vi "Day6Part2.vi"(11 "Input":string="47|53\n97|13\n97|61\n97|47\n75|29\n61|13\n75|53\n29|13\n97|29\n53|29\n61|53\n97|53\n61|29\n47|13\n75|47\n97|75\n47|61\n75|61\n47|29\n75|13\n53|13") -> (3 "Result":i64)   [LabVIEW 2024]
uses:
  <vilib>/Utility/miscctls.llb/LVMapReplaceAction.ctl
  <userlib>/_OpenG.lib/string/string.llb/openg_string.lvlib
panel:
  out "Array":bool[][](array[boolean])
  out "element":string
  out "X":i32
  out "Y":i32
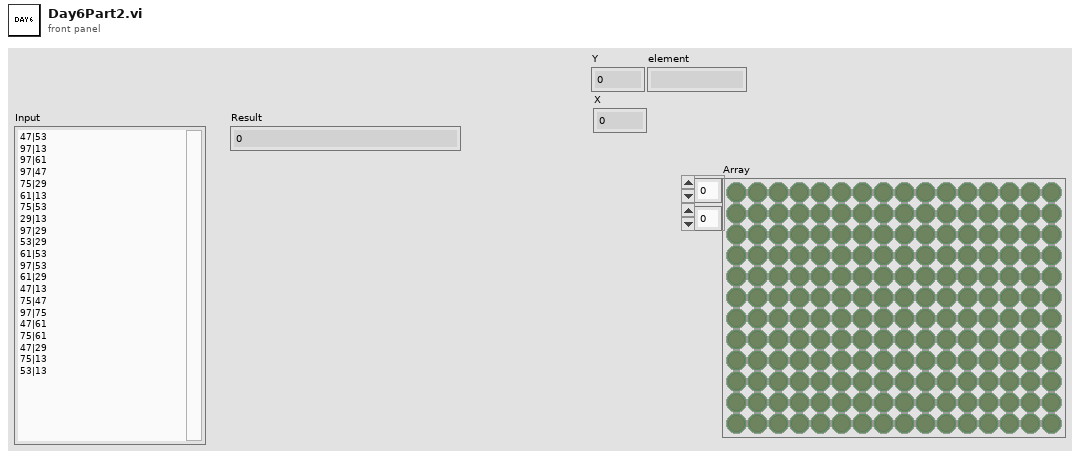
[diagram p1: front panel]
types:
  T1 = typedef "LVMapReplaceAction.ctl" = enum32{"Modify Entry only if found", "Add or Modify Entry", "Delete Entry"}
  T2 = map{cluster{i32, "offset past replacement":i32}, string[]}
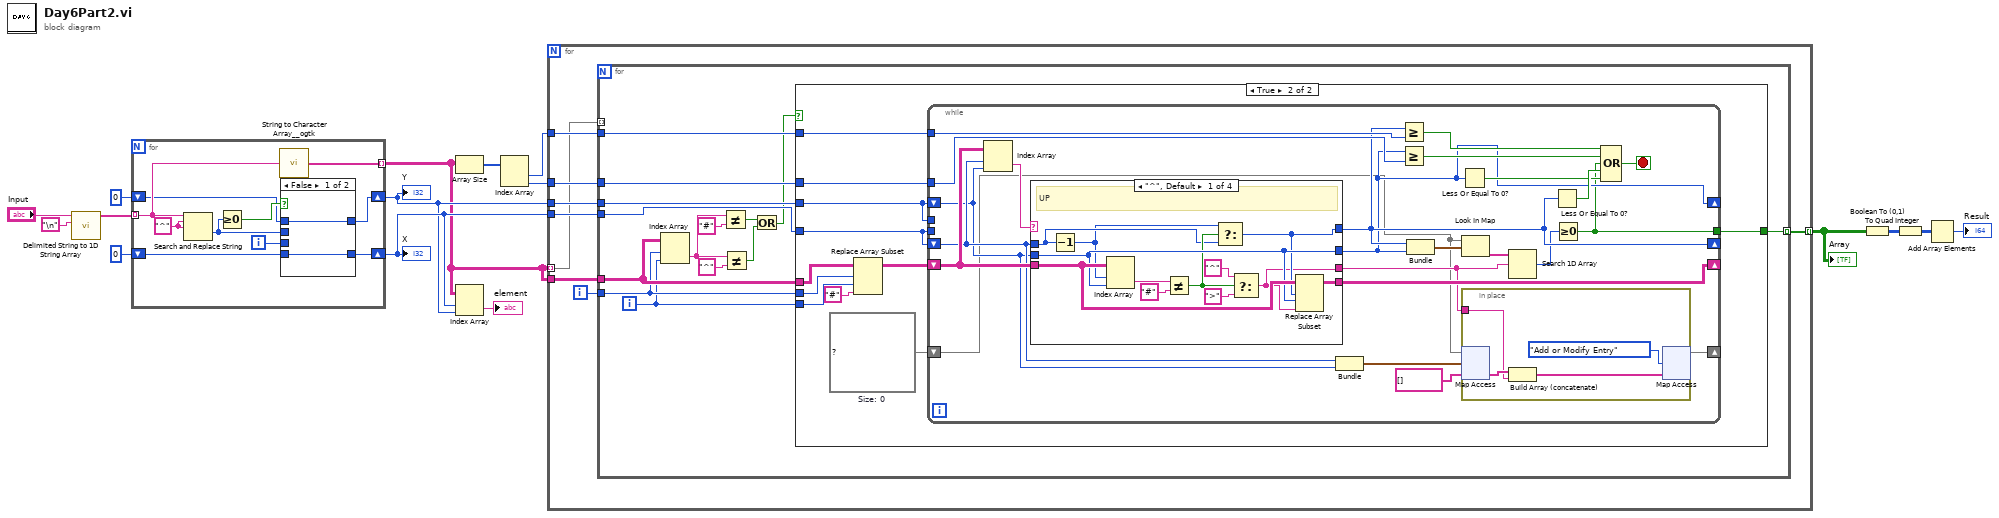
[diagram p0: block diagram]
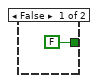
[diagram p2: hidden frame]
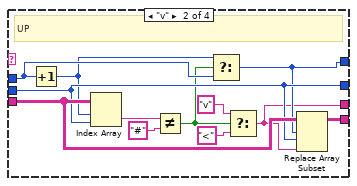
[diagram p3: hidden frame]
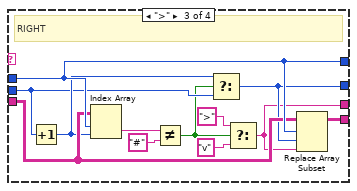
[diagram p4: hidden frame]
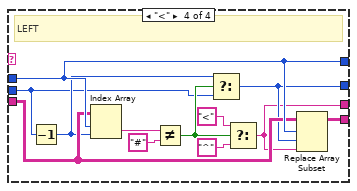
[diagram p5: hidden frame]
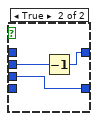
[diagram p6: hidden frame]
diagram:
  n1 = call <vilib>:"Delimited String to 1D String Array.vi"("delimiter"="\n", "delimited string"="Input") -> ("string array"=w14:string[])  [unwired: 9 in]
  n2 = for {
    tunnel: w14 -> [w25] mode=indexing
    tunnel: [w26] -> w4 mode=indexing
    shift-right: [w20] -> w8
    shift-left: 0 -> [w19]
    shift-right: [w18] -> w7
    shift-left: 0 ("offset past replacement") -> [w17]
    i -> [w21]
    w24 = "^" ("search string")
    n3 = Search and Replace String(input string=w25, search string=w24, replace string=w24) -> (offset past replacement=w22:i32)  [unwired: 5 in, 3 out]
    n4 = Greater Or Equal To 0?(x=w22) -> (x >= 0?=w23:bool)
    n5 = call <userlib>:"String to Character Array__ogtk.vi"("Input String"=w25) -> ("Character Array"=w26:string[])
    n6 = case shown="False" w23 {
      tunnel: w22 -> [_ w30]
      tunnel: w21 -> [_ w31]
      tunnel: [w28 w31] -> w20
      tunnel: w19 -> [w28 _]
      tunnel: [w27 w29] -> w18
      tunnel: w17 -> [w27 _]
      frame False {
      }
      frame True {
        n7 = Decrement(x=w30) -> (x-1=w29:i32)
      }
    }
  }
  "Y" <- w7
  "X" <- w8
  n8 = Array Size(array=w4) -> (size(s)=w10:i32[])
  n9 = Index Array(array=w4, index (row)=w8, index (col)=w7) -> (element=→"element":string)
  n10 = Index Array(array=w10) -> (element #1=w6:i32, element #2=w5:i32)  [unwired: 2 in]
  n11 = for {
    tunnel: w4 -> [w35] mode=indexing
    tunnel: w8 -> [w39]
    tunnel: w7 -> [w38]
    tunnel: w6 -> [w37]
    tunnel: w5 -> [w36]
    tunnel: w4 -> [w34]
    tunnel: [w32] -> w3 mode=indexing
    i -> [w33]
    n12 = for {
      tunnel: w39 -> [w53]
      tunnel: w38 -> [w52]
      tunnel: w37 -> [w51]
      tunnel: w36 -> [w50]
      tunnel: w35 -> [_] mode=indexing
      tunnel: w34 -> [w49]
      tunnel: w33 -> [w41]
      tunnel: [w42] -> w32 mode=indexing
      i -> [w40]
      n13 = Index Array(array=w49, index (row)=w41, index (col)=w40) -> (element=w47:string)
      n14 = Not Equal?(x=w47, y="#") -> (x != y?=w45:bool)
      n15 = Not Equal?(x=w47, y="^") -> (x != y?=w44:bool)
      n16 = Or(x=w45, y=w44) -> (x .or. y?=w43:bool)
      n17 = case shown="True" w43 {
        tunnel: w53 -> [_ w57]
        tunnel: w52 -> [_ w56]
        tunnel: w51 -> [_ w65]
        tunnel: w50 -> [_ w64]
        tunnel: w49 -> [_ w62]
        tunnel: [FALSE w61] -> w42
        tunnel: w41 -> [_ w60]
        tunnel: w40 -> [_ w59]
        frame False {
        }
        frame True {
          w55 = T2 {}  # Size: 0
          n18 = Replace Array Subset(array=w62, new element="#" ("new element/subarray"), index (row)=w60, index (col)=w59) -> (w63:string[][])
          n19 = while {
            shift-right: [w73] -> _
            shift-left: w57 -> [w78]
            shift-right: [w72] -> _
            shift-left: w56 -> [w77]
            shift-right: [w86] -> _
            shift-left: w63 -> [w87]
            tunnel: w65 -> [w85]
            tunnel: w64 -> [w84]
            tunnel: [w67] -> w61
            tunnel: w57 -> [_]
            tunnel: w56 -> [_]
            shift-right: [w74] -> _
            shift-left: w55 -> [w66]
            stop <- w81 stop-if-true
            n20 = Index Array(array=w87, index (row)=w78, index (col)=w77) -> (element=w88:string)
            n21 = case shown="\"^\", Default" w88 {
              tunnel: w78 -> [w97 w110 w128 w140]
              tunnel: [w95 w108 w128 w140] -> w73
              tunnel: w77 -> [w102 w114 w121 w132]
              tunnel: [w102 w114 w120 w131] -> w72
              tunnel: w87 -> [w103 w115 w126 w138]
              tunnel: [w99 w111 w123 w135] -> w86
              tunnel: [w93 w105 w117 w129] -> w69
              frame "^", Default {
                # "UP"
                n22 = Decrement(x=w97) -> (x-1=w96:i32)
                n23 = Index Array(array=w103, index (row)=w96, index (col)=w102) -> (element=w94:string)
                n24 = Not Equal?(x=w94, y="#") -> (x != y?=w98:bool)
                n25 = Select(t=w96, s=w98, f=w97) -> (s? t:f=w95:i32)
                n26 = Select(t="^", s=w98, f=">") -> (s? t:f=w93:string)
                n27 = Replace Array Subset(array=w103, new element=w93, index (row)=w95, index (col)=w102) -> (w99:string[][])
              }
              frame "v" {
                # "UP"
                n28 = Increment(x=w110) -> (x+1=w109:i32)
                n29 = Index Array(array=w115, index (row)=w109, index (col)=w114) -> (element=w106:string)
                n30 = Not Equal?(x=w106, y="#") -> (x != y?=w107:bool)
                n31 = Select(t=w109, s=w107, f=w110) -> (s? t:f=w108:i32)
                n32 = Select(t="v", s=w107, f="<") -> (s? t:f=w105:string)
                n33 = Replace Array Subset(array=w115, new element=w105, index (row)=w108, index (col)=w114) -> (w111:string[][])
              }
              frame ">" {
                # "RIGHT"
                n34 = Increment(x=w121) -> (x+1=w122:i32)
                n35 = Index Array(array=w126, index (row)=w128, index (col)=w122) -> (element=w118:string)
                n36 = Not Equal?(x=w118, y="#") -> (x != y?=w119:bool)
                n37 = Select(t=w122, s=w119, f=w121) -> (s? t:f=w120:i32)
                n38 = Select(t=">", s=w119, f="v") -> (s? t:f=w117:string)
                n39 = Replace Array Subset(array=w126, new element=w117, index (row)=w128, index (col)=w120) -> (w123:string[][])
              }
              frame "<" {
                # "LEFT"
                n40 = Decrement(x=w132) -> (x-1=w133:i32)
                n41 = Index Array(array=w138, index (row)=w140, index (col)=w133) -> (element=w130:string)
                n42 = Not Equal?(x=w130, y="#") -> (x != y?=w134:bool)
                n43 = Select(t=w133, s=w134, f=w132) -> (s? t:f=w131:i32)
                n44 = Select(t="<", s=w134, f="^") -> (s? t:f=w129:string)
                n45 = Replace Array Subset(array=w138, new element=w129, index (row)=w140, index (col)=w131) -> (w135:string[][])
              }
            }
            n46 = Bundle(w78, "offset past replacement"=w77) -> (w76:cluster{i32, "offset past replacement":i32})  [unwired: 1 in]
            n47 = Greater Or Equal?(x=w73, y=w85) -> (x >= y?=w83:bool)
            n48 = Greater Or Equal?(x=w72, y=w84) -> (x >= y?=w82:bool)
            n49 = Bundle(w73, "offset past replacement"=w72) -> (w71:cluster{i32, "offset past replacement":i32})  [unwired: 1 in]
            n50 = Less Or Equal To 0?(x=w72) -> (x <= 0?=w79:bool)
            n51 = Look In Map(map=w66, key=w71) -> (value=w70:string[])  [unwired: 1 in, 1 out]
            n52 = in-place {
              in-place-border: w69 -> [w91]
              n53 = in-place-map #1(w66, w76, string[] []) -> (w92:string[])  [unwired: 1 out]
              n54 = Build Array (concatenate)(w92, w91) -> (w90:string[])
              n55 = in-place-map #1(w90, LVMapReplaceAction."Add or Modify Entry" ("action")) -> (w74:T2)  [unwired: 2 out]
            }
            n56 = Search 1D Array(1D array=w70, element=w69) -> (index of element=w68:i32)  [unwired: 1 in]
            n57 = Less Or Equal To 0?(x=w73) -> (x <= 0?=w80:bool)
            n58 = Greater Or Equal To 0?(x=w68) -> (x >= 0?=w67:bool)
            n59 = Compound Arithmetic op=OR(w83, w82, w67, w80, w79) -> (w81:bool)
          }
        }
      }
    }
  }
  "Array" <- w3
  n60 = Boolean To (0,1)(Boolean=w3) -> (0, 1=w2:i16[][])
  n61 = To Quad Integer(1:w2) -> (0:w1:i64[][])
  n62 = Add Array Elements(numeric array=w1) -> (sum=→"Result":i64)
